vi "Slam Test.vi"() -> ()   [LabVIEW 2017]
uses:
  <vilib>/robotics/Steering/Wheel/Wheel Parameters.ctl
  <vilib>/robotics/Steering/Wheel/Rotation Direction.ctl
  <vilib>/Platform/TimedLoop/XDataNode/timing_clust.ctl
  <vilib>/Platform/TimedLoop/XDataNode/nitl_modes.ctl
  <vilib>/Platform/TimedLoop/XDataNode/wakeup.ctl
  <vilib>/robotics/Steering/Fixed Wheel/NI_Robotics_Fixed Wheel.lvclass
  C:/Program Files (x86)/National Instruments/LabVIEW 2017/vi.lib/robotics/Steering/Wheel/NI_Robotics_Wheel.lvclass
  <vilib>/robotics/Steering/Fixed Wheel/Create Fixed Wheel.vi
  <vilib>/robotics/Steering/Steering Frame/Create User Defined Steering Frame.vi
  <vilib>/robotics/Steering/Create Steering Frame/NI_Robotics_Create Steering Frame.xnode
  <vilib>/robotics/Steering/Class Type Definitions/Steering Frame.ctl
  <vilib>/Platform/TimedLoop/XDataNode/XDataNode.xnode
  <vilib>/Platform/TimedLoop/XDataNode/XDNodeRunTimeDep.lvlib
  Globals/Gyro.vi
  <vilib>/robotics/Steering/Steering Frame/NI_Robotics_Steering Frame.lvclass
  <vilib>/robotics/Steering/Class Type Definitions/NI_Robotics_Steering Class Types.lvlib
  <vilib>/robotics/Steering/Wheel/NI_Robotics_Wheel.lvclass
  <vilib>/robotics/Steering/Steering Frame/Apply Steering Frame Velocity to Motors.vi
panel:
  in  "Lidar Offset (mm)":dbl=-100.0 format="%#_13g"
  out "GYRO IS FUCKED":bool
  out "Estimated Pose (Degrees)":cluster{"X":dbl, "Y":dbl, "R":dbl}
  in  "Desired Velocity":dbl[](array[numeric])=[0.0, 0.0, 0.0]
  out "Gyro Bias":cluster{"X":dbl, "Y":dbl, "Z":dbl}={"X"=0.039458598891488325, "Y"=-0.012762257416847495, "Z"=-0.06349169800034307}
  out "slam run time":u32
  out "Estimated Pose":cluster{"X":dbl, "Y":dbl, "R":dbl}
  in  "slam itearations":i32=4
  out "Intensity Graph":u16[][](graph)
  out "stopping":bool
  out "libslam works":bool
  in  "stop":bool
  out "XY Graph":cluster{"X":dbl[], "Y":dbl[]}[](graph)
  out "lidar run time":u32
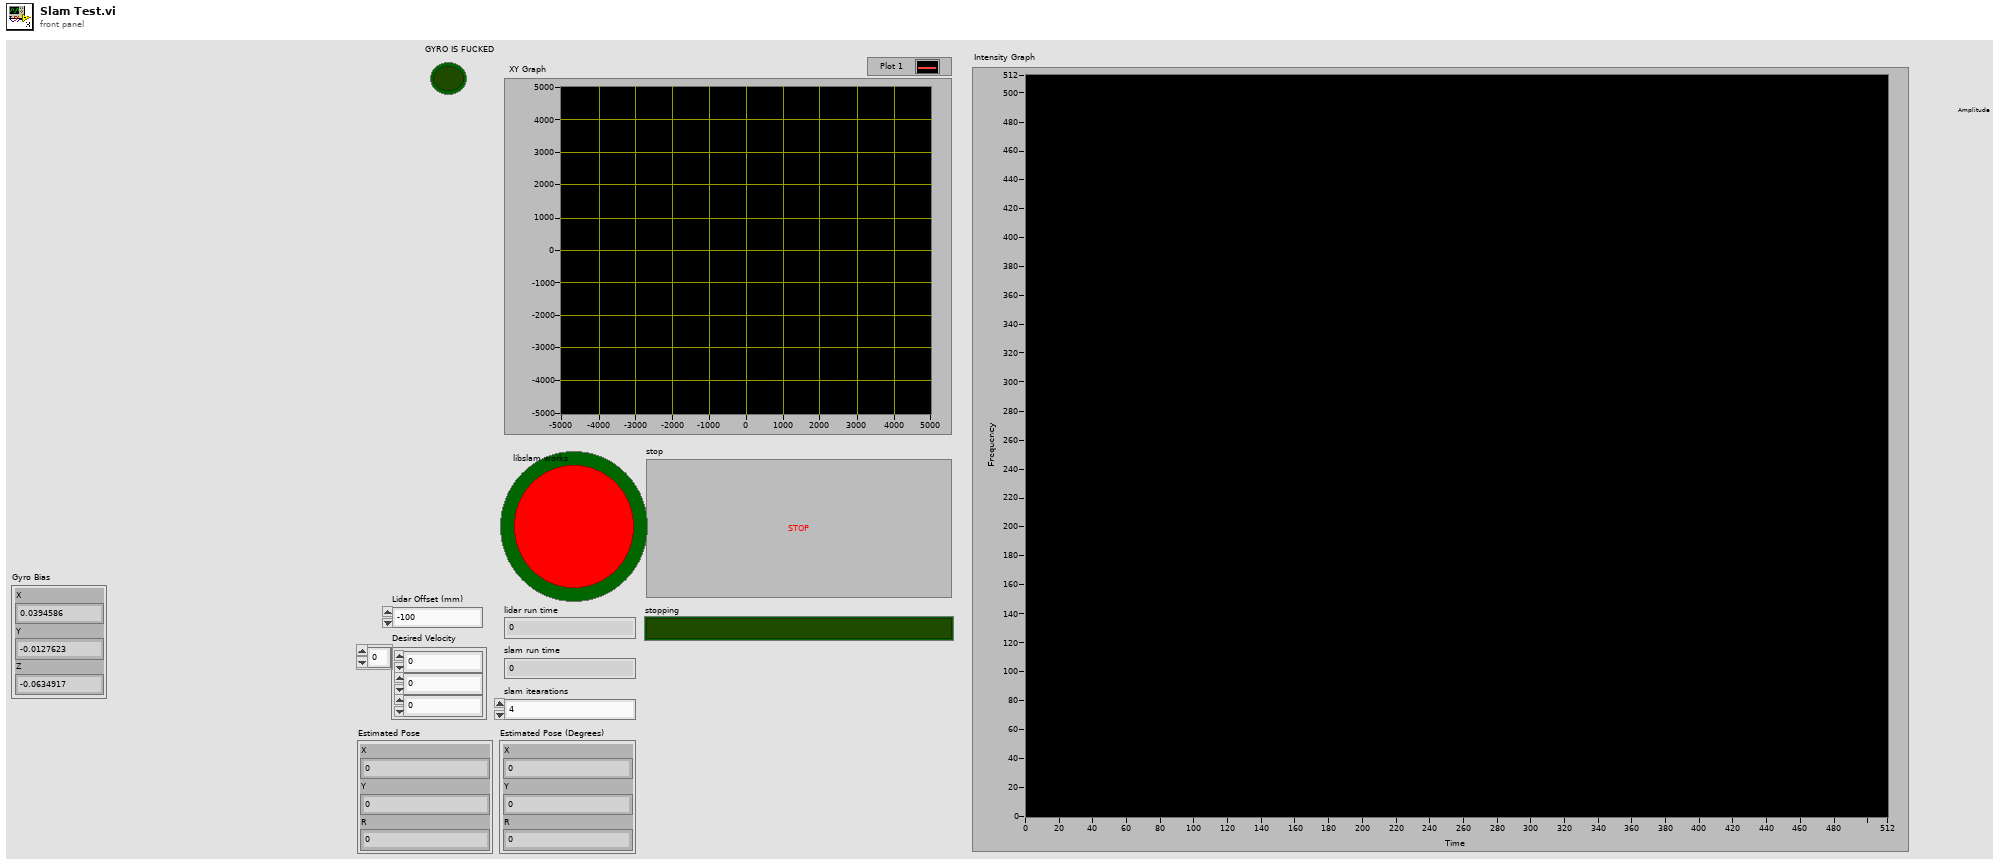
[diagram p1: front panel]
types:
  T1 = cluster{dbl[], dbl[], "Estimated Pose Delta":cluster{"X":dbl, "Y":dbl, "R":dbl}}
  T2 = typedef "NI_Robotics_Wheel.lvclass/Wheel Parameters.ctl" = cluster{"wheel radius":dbl, "gear ratio":dbl, "forward rotation direction":T3}
  T3 = typedef "NI_Robotics_Wheel.lvclass/Rotation Direction.ctl" = u16
  T4 = typedef "XDNodeRunTimeDep.lvlib/timing_clust.ctl" = cluster{"Expected End [f-1]":u64, "Actual End [f-1]":u64, "Finished Late? [f-1]":bool, "Expected End [i-1]":u64, "Actual End [i-1]":u64, "Finished Late? [i-1]":bool, "Expected Start [i]":u64, "Actual Start [i]":u64, "Expected Start [f]":u64, "Actual Start [f]":u64, "Source Name":string, "Structure Name":string, "Period":i64, "Deadline":i64, "Offset":i64, "Start":i64, "Priority":i32, "Timeout":i32, "Mode":T5, "Wakeup Reason":T6, "Error":errorcluster, "Source Type":string, "Secondary Source Type":string, "Global End Time":u64, "Global Start Time":u64, "Frame Duration":u64, "Iteration Duration":u64, "Assigned CPU":i32, "I/O Scan Engine Mode":u32}
  T5 = typedef "XDNodeRunTimeDep.lvlib/nitl_modes.ctl" = enum32{"No Change", "Process missed periods, maintain original phase", "Discard missed periods, maintain original phase", "Process missed periods, ignore original phase", "Discard missed periods, ignore original phase"}
  T6 = typedef "XDNodeRunTimeDep.lvlib/wakeup.ctl" = enum32{"Normal", "Aborted", "Asynchronous wakeup", "Timing source error", "Timed loop error", "Timeout"}
  T7 = typedef "I2C.lvlib/I2C Reference.ctl" = cluster{"myRIO Reference":T8, "I2C Channels Enum":T12, "I2C Configuration":T13}
  T8 = typedef "myRIO Generic Hardware Reference.ctl" = cluster{"myRIO Model":T9, "myRIO Hardware Reference":T10}
  T9 = typedef "Hardware Version Enum.ctl" = enum16{"Unknown", "myRIO-1900", "myRIO-1950", "roboRIO", "NI ELVIS RIO CM"}
  T10 = typedef "myRIO v1.0 Reference.ctl" = cluster{"Generic FPGA Reference":T11, "Allow multiple opens":bool}
  T11 = typedef "Generic FPGA Reference.ctl" = refnum<k20>
  T12 = typedef "I2C Channels Enum.ctl" = enum16{"Not Connected", "A/I2C", "B/I2C", "I2C/I2C"}
  T13 = typedef "I2C.lvlib/I2C Configuration.ctl" = cluster{"I2C Transfer Rate":T14}
  T14 = typedef "I2C.lvlib/I2C Transfer Rate.ctl" = enum16{"Standard mode (100 kbps)", "Fast mode (400 kbps)"}
  T15 = typedef "NI_Robotics_Steering Class Types.lvlib/Steering Frame.ctl" = refnum<class "NI_Robotics_Steering Frame.lvclass">
  T16 = cluster{"X":dbl[], "Y":dbl[], "Estimated Pose":cluster{"X":dbl, "Y":dbl, "R":dbl}}
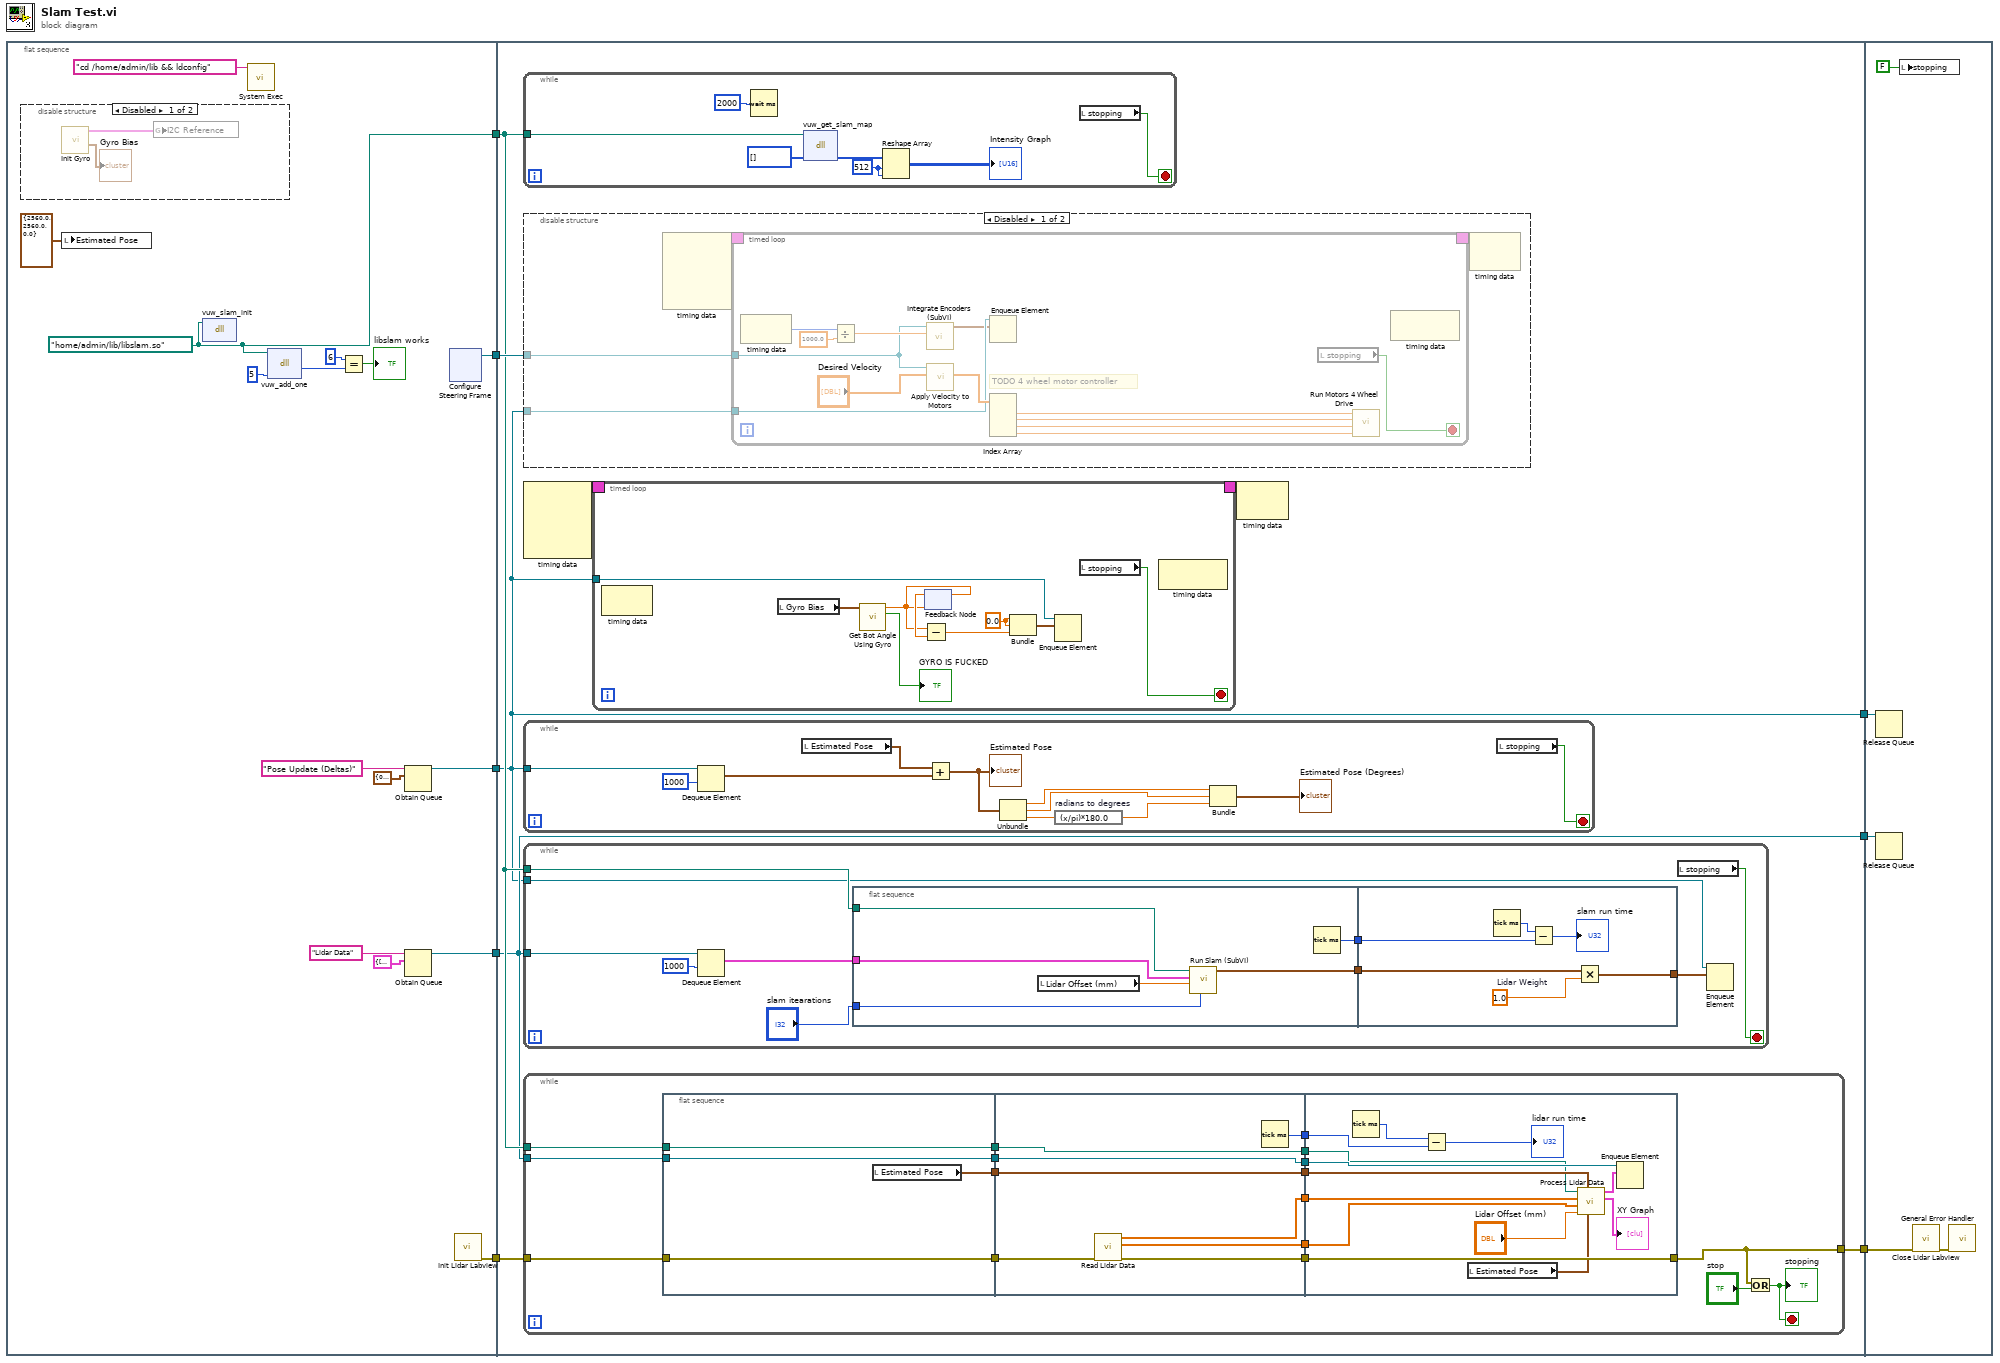
[diagram p0: block diagram]
diagram:
  n1 = flat-sequence {
    tunnel: [w22] -> w7
    tunnel: [w13] -> w6
    tunnel: [w18] -> w5
    tunnel: [w17] -> w4
    tunnel: [w15] -> w3
    tunnel: [w56] -> w8
    tunnel: w7 -> [w55]
    tunnel: w6 -> [w53]
    tunnel: w5 -> [w50]
    tunnel: w4 -> [w54]
    tunnel: w3 -> [w49]
    tunnel: [w50] -> w2
    tunnel: [w49] -> w1
    tunnel: w8 -> [w177]
    tunnel: w2 -> [w176]
    tunnel: w1 -> [w174]
    frame #0 {
      w13 = path "/home/admin/lib/libslam.so" ("path in")
      n2 = disable-structure shown="Disabled" {
        frame Disabled {
          n3 = call "Init Gyro.vi"() -> ("Gyro Bias"=→"Gyro Bias":cluster{"X":dbl, "Y":dbl, "Z":dbl}, "I2C Ref Out"=w25:T7)  [unwired: 9 in, 1 out]
          n4 = global write "Gyro.vi" "I2C Reference"(w25) -> ()
        }
        frame Enabled {
        }
      }
      n5 = local write "Estimated Pose"(cluster{"X":dbl, "Y":dbl, "R":dbl} {"X"=2560.0, "Y"=2560.0, "R"=0.0} ("Estimated Pose")) -> ()
      n6 = dll-call lib="home/admin/lib/libslam.so" fn="vuw_slam_init"(path in=w13) -> ()  [unwired: 3 in, 2 out]
      n7 = call <vilib>:"System Exec.vi"("command line"="cd /home/admin/lib && ldconfig") -> ()  [unwired: 7 in, 4 out]
      n8 = dll-call lib="home/admin/lib/libslam.so" fn="vuw_add_one"(path in=w13, "x"=5) -> ("return type"=w12:i32)  [unwired: 3 in, 2 out]
      n9 = Equal?(x=6, y=w12) -> (x = y?=→"libslam works":bool)
      n10 = Obtain Queue(name (unnamed)="Pose Update (Deltas)", element data type=cluster{"X":dbl, "Y":dbl, "R":dbl} {"X"=0.0, "Y"=0.0, "R"=0.0} ("Estimated Pose Delta")) -> (queue out=w15:refnum<queue>)  [unwired: 3 in, 2 out]
      n11 = Obtain Queue(name (unnamed)="Lidar Data", element data type=T1 {[], [], "Estimated Pose Delta"={"X"=0.0, "Y"=0.0, "R"=0.0}} ("output cluster")) -> (queue out=w18:refnum<queue>)  [unwired: 3 in, 2 out]
      n12 = xnode ("Configure Steering Frame")() -> ("steering frame out"=w22:T15)  [unwired: 1 in, 1 out]
      n13 = call "Init Lidar Labview.vi"() -> ("error out"=w17:errorcluster)  [unwired: 11 in]
    }
    frame #1 {
      n14 = while {
        tunnel: w53 -> [w125]
        stop <- w126 stop-if-true
        w130 = 512 ("dimension size")
        n15 = Wait (ms)(milliseconds to wait=u32 2000) -> ()  [unwired: 1 out]
        n16 = dll-call lib="home/admin/lib/libslam.so" fn="vuw_get_slam_map"(path in=w125, "map"=u16[] []) -> ("map"=w131:u16[])  [unwired: 3 in, 2 out]
        n17 = Reshape Array(w131, w130, w130) -> (→"Intensity Graph":u16[][])
        n18 = local read "stopping"() -> (w126:bool)
      }
      n19 = disable-structure shown="Disabled" {
        disable-tunnel: w55 -> [w71 _]
        disable-tunnel: w49 -> [w70 _]
        frame Disabled {
          n20 = node-c288() -> (w73:T4)  [unwired: 4 in]
          n21 = timed-loop {
            timing: w73 -> [_]
            timing-out: [_] -> w72
            tunnel: w71 -> [w79]
            tunnel: w70 -> [w75]
            stop <- w86 stop-if-true
            # "TODO 4 wheel motor controller"
            n22 = node-c288() -> (w83:i64)  [unwired: 1 in]
            n23 = Divide(x=w83, y=1000.0) -> (x/y=w84:dbl)
            n24 = call "Integrate Encoders (SubVI).vi"("dt"=w84, "NI_Robotics_Steering Frame in"=w79) -> ("Estimated Pose Delta"=w74:cluster{dbl, dbl, dbl})  [unwired: 9 in]
            n25 = call-poly <vilib>:"Apply Velocity to Motors.vi"("steering frame velocity"="Desired Velocity", "steering frame in"=w79) -> ("ccw motor velocity setpoints"=w81:dbl[])  [unwired: 5 in, 4 out]
            n26 = Enqueue Element(queue=w75, element=w74) -> ()  [unwired: 2 in, 3 out]
            n27 = Index Array(array=w81) -> (element #1=w82:dbl, element #2=w78:dbl, element #3=w77:dbl, element #4=w76:dbl)  [unwired: 4 in]
            n28 = local read "stopping"() -> (w86:bool)
            n29 = call "Run Motors 4 Wheel Drive.vi"("Back Right"=w76, "Front Right"=w77, "Back Left"=w78, "Front Left"=w82) -> ()  [unwired: 8 in]
            n30 = node-c288() -> ()  [unwired: 1 in, 1 out]
          }
          n31 = node-c288(w72) -> ()  [unwired: 1 out]
        }
        frame Enabled {
        }
      }
      n32 = node-c288() -> (w52:T4)  [unwired: 4 in]
      n33 = while {
        tunnel: w49 -> [w100]
        stop <- w102 stop-if-true
        n34 = Dequeue Element(queue=w100, timeout in ms (-1)=1000) -> (element=w98:cluster{"X":dbl, "Y":dbl, "R":dbl})  [unwired: 1 in, 3 out]
        n35 = local read "Estimated Pose"() -> (w99:cluster{"X":dbl, "Y":dbl, "R":dbl})
        n36 = Add(x=w99, y=w98) -> (x+y=w97:cluster{"X":dbl, "Y":dbl, "R":dbl})
        "Estimated Pose" <- w97
        n37 = Unbundle(w97) -> ("X"=w96:dbl, "Y"=w95:dbl, "R"=w94:dbl)
        n38 = expression code="(x/pi)*180.0" "radians to degrees"(w94) -> (w93:dbl)
        n39 = Bundle("X"=w96, "Y"=w95, "R"=w93) -> (→"Estimated Pose (Degrees)":cluster{"X":dbl, "Y":dbl, "R":dbl})  [unwired: 1 in]
        n40 = local read "stopping"() -> (w102:bool)
      }
      n41 = while {
        tunnel: w53 -> [w110]
        tunnel: w50 -> [w109]
        tunnel: w49 -> [w106]
        stop <- w112 stop-if-true
        n42 = Dequeue Element(queue=w109, timeout in ms (-1)=1000) -> (element=w111:T1)  [unwired: 1 in, 3 out]
        n43 = flat-sequence {
          tunnel: w111 -> [w118]
          tunnel: w110 -> [w117]
          tunnel: "slam itearations" -> [w116]
          tunnel: [w115] -> w104
          tunnel: [w114] -> w103
          tunnel: [w121] -> w105
          tunnel: w104 -> [w119]
          tunnel: w103 -> [w124]
          frame #0 {
            n44 = local read "Lidar Offset (mm)"() -> (w113:dbl)
            n45 = call "Run Slam (SubVI).vi"("slam itearations"=w116, "Lidar Offset from Center of Rotation (mm)"=w113, "Lidar Data"=w118, "Library Path"=w117) -> ("Pose Delta"=w115:cluster{"X":dbl, "Y":dbl, "R":dbl})  [unwired: 7 in]
            n46 = Tick Count (ms)() -> (millisecond timer value=w114:u32)
          }
          frame #1 {
            w120 = 1.0  # Lidar Weight
            n47 = Tick Count (ms)() -> (millisecond timer value=w123:u32)
            n48 = Subtract(x=w123, y=w124) -> (x-y=→"slam run time":u32)
            n49 = Multiply(x=w119, y=w120) -> (x*y=w121:cluster{"X":dbl, "Y":dbl, "R":dbl})
          }
        }
        n50 = local read "stopping"() -> (w112:bool)
        n51 = Enqueue Element(queue=w106, element=w105) -> ()  [unwired: 2 in, 3 out]
      }
      n52 = while {
        tunnel: [w144] -> w56
        tunnel: w54 -> [w141]
        tunnel: w50 -> [w138]
        tunnel: w53 -> [w133]
        stop <- w148 stop-if-true
        n53 = flat-sequence {
          tunnel: [w152] -> w142
          tunnel: w141 -> [w152]
          tunnel: [w151] -> w139
          tunnel: w138 -> [w150]
          tunnel: [w150] -> w137
          tunnel: [w149] -> w134
          tunnel: w133 -> [w149]
          tunnel: [w160] -> w146
          tunnel: [w159] -> w145
          tunnel: [w156] -> w143
          tunnel: w142 -> [w157]
          tunnel: [w158] -> w140
          tunnel: w139 -> [w158]
          tunnel: w137 -> [w155]
          tunnel: [w155] -> w136
          tunnel: [w154] -> w135
          tunnel: w134 -> [w154]
          tunnel: [w153] -> w132
          tunnel: w146 -> [w166]
          tunnel: w145 -> [w167]
          tunnel: [w173] -> w144
          tunnel: w143 -> [w173]
          tunnel: w140 -> [w172]
          tunnel: w136 -> [w169]
          tunnel: w135 -> [w168]
          tunnel: w132 -> [w162]
          frame #0 {
            n54 = local read "Estimated Pose"() -> (w151:cluster{"X":dbl, "Y":dbl, "R":dbl})
          }
          frame #1 {
            n55 = call "Read Lidar Data.vi"("error in (no error)"=w157) -> ("error out"=w156:errorcluster, "Direction"=w159:dbl[], "Magnitude"=w160:dbl[])  [unwired: 8 in]
            n56 = Tick Count (ms)() -> (millisecond timer value=w153:u32)
          }
          frame #2 {
            n57 = Tick Count (ms)() -> (millisecond timer value=w163:u32)
            n58 = Subtract(x=w163, y=w162) -> (x-y=→"lidar run time":u32)
            n59 = local read "Estimated Pose"() -> (w170:cluster{"X":dbl, "Y":dbl, "R":dbl})
            n60 = call "Process Lidar Data.vi"("Estimated Pose After Scan"=w170, "Estimated Pose Before Scan"=w172, "Lidar Offset from Center of Rotation (mm)"="Lidar Offset (mm)", "Direction"=w167, "Magnitude"=w166, "path in"=w168) -> ("Data Comparison"=→"XY Graph":cluster{"X":dbl[], "Y":dbl[]}[], "Lidar Scan"=w171:T16)  [unwired: 4 in]
            n61 = Enqueue Element(queue=w169, element=w171) -> ()  [unwired: 2 in, 3 out]
          }
        }
        n62 = Or(x=w144, y="stop") -> (x .or. y?=w148:bool)
        "stopping" <- w148
      }
      n63 = timed-loop {
        timing: w52 -> [_]
        timing-out: [_] -> w51
        tunnel: w49 -> [w63]
        stop <- w62 stop-if-true
        w57 = 0.0 ("x-y")
        n64 = node-c288() -> ()  [unwired: 1 in, 1 out]
        n65 = local read "Gyro Bias"() -> (w65:cluster{"X":dbl, "Y":dbl, "Z":dbl})
        n66 = call "Get Bot Angle Using Gyro.vi"("Gyro bias"=w65) -> ("GYRO IS FUCKED"=→"GYRO IS FUCKED":bool, "Z Rotation (rads)"=w60:dbl)  [unwired: 9 in]
        n67 = feedback-in #1(w60) -> ()
        n68 = feedback #1(w60) -> (w61:dbl)
        n69 = Subtract(x=w60, y=w61) -> (x-y=w59:dbl)
        n70 = Bundle("x-y"=w57, "x-y"=w57, w59) -> (w58:cluster{"x-y":dbl, "x-y":dbl, dbl})  [unwired: 1 in]
        n71 = Enqueue Element(queue=w63, element=w58) -> ()  [unwired: 2 in, 3 out]
        n72 = local read "stopping"() -> (w62:bool)
        n73 = node-c288() -> ()  [unwired: 1 in, 1 out]
      }
      n74 = node-c288(w51) -> ()  [unwired: 1 out]
    }
    frame #2 {
      n75 = Release Queue(queue=w174) -> ()  [unwired: 2 in, 3 out]
      n76 = Release Queue(queue=w176) -> ()  [unwired: 2 in, 3 out]
      n77 = local write "stopping"(FALSE) -> ()
      n78 = call "Close Lidar Labview.vi"("error in (no error)"=w177) -> ("error out"=w178:errorcluster)  [unwired: 10 in]
      n79 = call <vilib>:"General Error Handler.vi"("error in (no error)"=w178) -> ()  [unwired: 10 in, 5 out]
    }
  }
